vi "PhotonTrackedTarget_New.vi"(0 "Pitch":dbl, 1 "Yaw":dbl, 3 "Fiducial Id":i32, 5 "Area":dbl, 7 "Skew":dbl, 10 "DetectedCorners":T1[](array[typedef]), 12 "BestCameraToTarget":T2={"TRANSLATION3D"={"X"=0.0, "Y"=0.0, "Z"=0.0}, "ROTATION3D"={"Q_quaternion"={"R"=1.0, "V"=[0.0, 0.0, 0.0]}}, "XF"=FALSE} {"TRANSLATION3D"."Z" format="%14.3f"; "TRANSLATION3D"."Y" format="%14.3f"; "TRANSLATION3D"."X" format="%14.3f"}, 13 "AltCameraToTarget":T2={"TRANSLATION3D"={"X"=0.0, "Y"=0.0, "Z"=0.0}, "ROTATION3D"={"Q_quaternion"={"R"=1.0, "V"=[0.0, 0.0, 0.0]}}, "XF"=FALSE} {"TRANSLATION3D"."Z" format="%14.3f"; "TRANSLATION3D"."Y" format="%14.3f"; "TRANSLATION3D"."X" format="%14.3f"}, 14 "MinAreaRectCorners":T1[](array[typedef]), 15 "Pose Ambiguity":dbl) -> (4 "TrackedTarget":T6={"Yaw"=0.0, "Pitch"=0.0, "Area"=0.0, "Skew"=0.0, "MinAreaRectCorners"=[], "BestCameraToTarget"={"TRANSLATION3D"={"X"=0.0, "Y"=0.0, "Z"=0.0}, "ROTATION3D"={"Q_quaternion"={"R"=1.0, "V"=[0.0, 0.0, 0.0]}}, "XF"=FALSE}, "FiducialId"=0, "AltCameraToTarget"={"TRANSLATION3D"={"X"=0.0, "Y"=0.0, "Z"=0.0}, "ROTATION3D"={"Q_quaternion"={"R"=1.0, "V"=[0.0, 0.0, 0.0]}}, "XF"=FALSE}, "PoseAmbiguity"=0.0, "DetectedCorners"=[], "ObjDetectId"=0, "ObjDetectConf"=0.0} {"AltCameraToTarget"."TRANSLATION3D"."Z" format="%14.3f"; "AltCameraToTarget"."TRANSLATION3D"."Y" format="%14.3f"; "AltCameraToTarget"."TRANSLATION3D"."X" format="%14.3f"; "BestCameraToTarget"."TRANSLATION3D"."Z" format="%14.3f"; "BestCameraToTarget"."TRANSLATION3D"."Y" format="%14.3f"; "BestCameraToTarget"."TRANSLATION3D"."X" format="%14.3f"})   [LabVIEW 2019, in "PhotonVisionLib.lvlib"]
doc: "Create a new TracedTarget data cluster\n\nInputs:\n - Yaw -- \n - Pitch -- \n - Area -- \n - Skew -- \n - CameraToTarget -- Transform2d\n - MinAreaRectCorners -- Array of 4 corners.\n - Pose Ambiguity\n - Fiducial ID\n - Detected Corners\n\nOutputs:\n - TrackedTarget -- Created TrackedTarget cluster."
uses:
  PhotonVisionLib.lvlib
  TypeDef/PhotonTrackedTargetType.ctl
  TypeDef/TargetCornerType.ctl
  <vilib>/Rock Robotics/WPI/ThirdParty/JAS_Junk/TrajLib/TypeDef/TRANSFORM3D.ctl
  <vilib>/Rock Robotics/WPI/ThirdParty/JAS_Junk/TrajLib/TypeDef/TRANSLATION3D.ctl
  <vilib>/Rock Robotics/WPI/ThirdParty/JAS_Junk/TrajLib/TypeDef/ROTATION3D.ctl
  <vilib>/Rock Robotics/WPI/ThirdParty/JAS_Junk/TrajLib/TypeDef/QUATERNION.ctl
  <vilib>/Rock Robotics/WPI/ThirdParty/JAS_Junk/TrajLib/Trajectory_Library.lvlib
panel:
  in  "DetectObjConf":sgl
  in  "ObjDetectId":i32
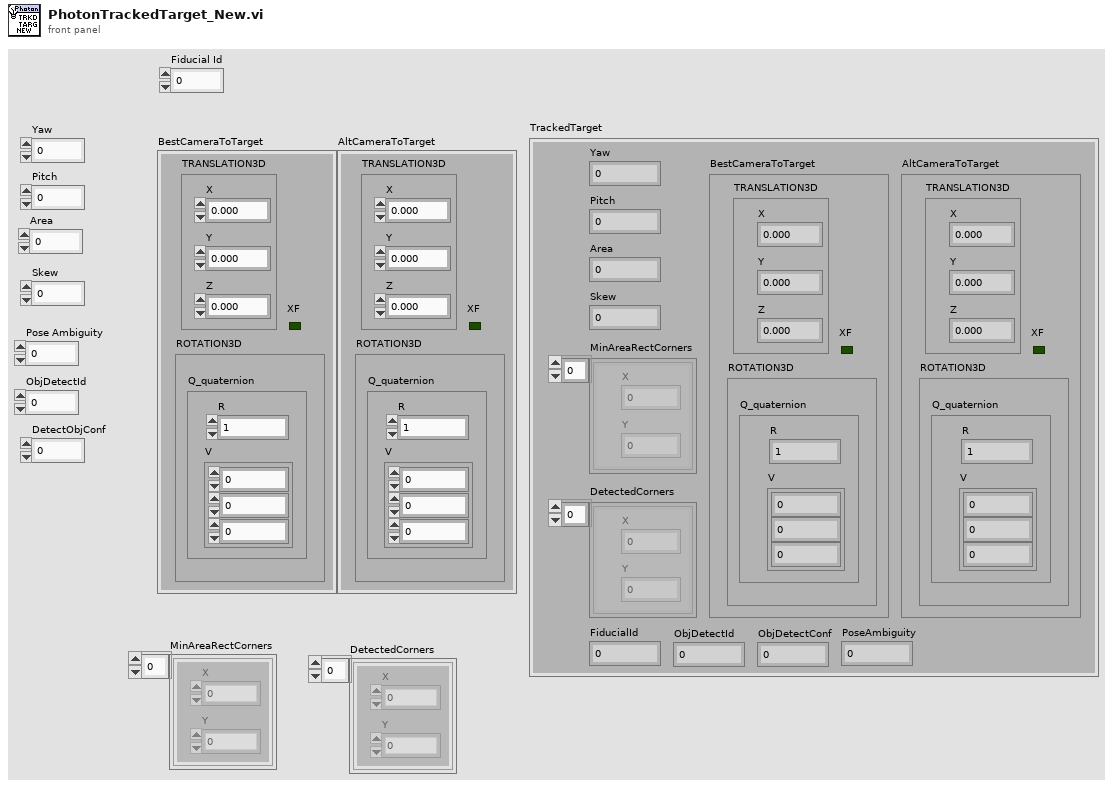
[diagram p1: front panel]
types:
  T1 = typedef "PhotonVisionLib.lvlib/TargetCornerType.ctl" = cluster{"X":dbl, "Y":dbl}
  T2 = typedef "Trajectory_Library.lvlib/TRANSFORM3D.ctl" = cluster{"TRANSLATION3D":T3, "ROTATION3D":T4, "XF":bool}
  T3 = typedef "Trajectory_Library.lvlib/TRANSLATION3D.ctl" = cluster{"X":dbl, "Y":dbl, "Z":dbl}
  T4 = typedef "Trajectory_Library.lvlib/ROTATION3D.ctl" = cluster{"Q_quaternion":T5}
  T5 = typedef "Trajectory_Library.lvlib/QUATERNION.ctl" = cluster{"R":dbl, "V":dbl[]}
  T6 = typedef "PhotonVisionLib.lvlib/PhotonTrackedTargetType.ctl" = cluster{"Yaw":dbl, "Pitch":dbl, "Area":dbl, "Skew":dbl, "MinAreaRectCorners":T1[], "BestCameraToTarget":T2, "FiducialId":i32, "AltCameraToTarget":T2, "PoseAmbiguity":dbl, "DetectedCorners":T1[], "ObjDetectId":i32, "ObjDetectConf":sgl}
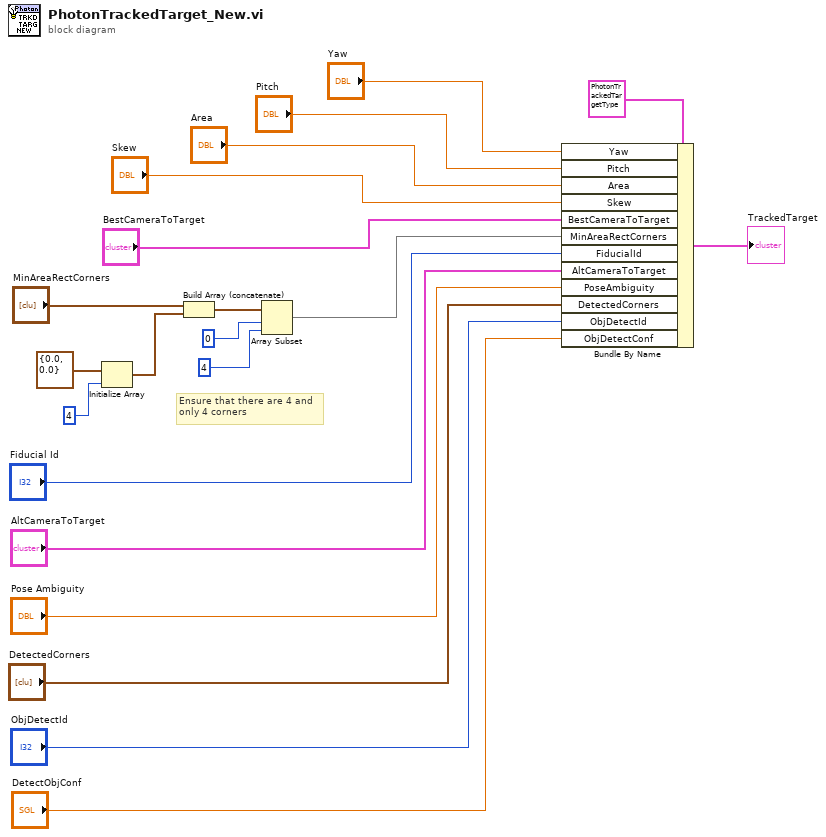
[diagram p0: block diagram]
diagram:
  # "Ensure that there are 4 and \nonly 4 corners"
  n1 = Initialize Array(T1 {"X"=0.0, "Y"=0.0} ("TargetCorner"), 4 ("dimension size")) -> (w11:T1[])
  n2 = Build Array (concatenate)("MinAreaRectCorners", w11) -> (w10:T1[])
  n3 = Array Subset(array=w10, index=0, length=4) -> (w7:T1[])
  n4 = Bundle By Name(cluster=T6 {"Yaw"=0.0, "Pitch"=0.0, "Area"=0.0, "Skew"=0.0, "MinAreaRectCorners"=[], "BestCameraToTarget"={"TRANSLATION3D"={"X"=0.0, "Y"=0.0, "Z"=0.0}, "ROTATION3D"={"Q_quaternion"={"R"=1.0, "V"=[0.0, 0.0, 0.0]}}, "XF"=FALSE}, "FiducialId"=0, "AltCameraToTarget"={"TRANSLATION3D"={"X"=0.0, "Y"=0.0, "Z"=0.0}, "ROTATION3D"={"Q_quaternion"={"R"=1.0, "V"=[0.0, 0.0, 0.0]}}, "XF"=FALSE}, "PoseAmbiguity"=0.0, "DetectedCorners"=[], "ObjDetectId"=0, "ObjDetectConf"=0.0} ("PhotonTrackedTarget"), "Yaw"="Yaw", "Pitch"="Pitch", "Area"="Area", "Skew"="Skew", "BestCameraToTarget"="BestCameraToTarget", "MinAreaRectCorners"=w7, "FiducialId"="Fiducial Id", "AltCameraToTarget"="AltCameraToTarget", "PoseAmbiguity"="Pose Ambiguity", "DetectedCorners"="DetectedCorners", "ObjDetectId"="ObjDetectId", "ObjDetectConf"="DetectObjConf") -> (→"TrackedTarget":T6)
